vi "ETH 6 Main.vi"(7 "ETH6 Q":refnum<queue>, 8 "error in (no error)":errorcluster, 11 "connection ID":refnum<k5>) -> (0 "error out 2":errorcluster, 3 "connection ID 2":refnum<k5>)   [LabVIEW 2022 SP3]
panel:
  in  "data in":string
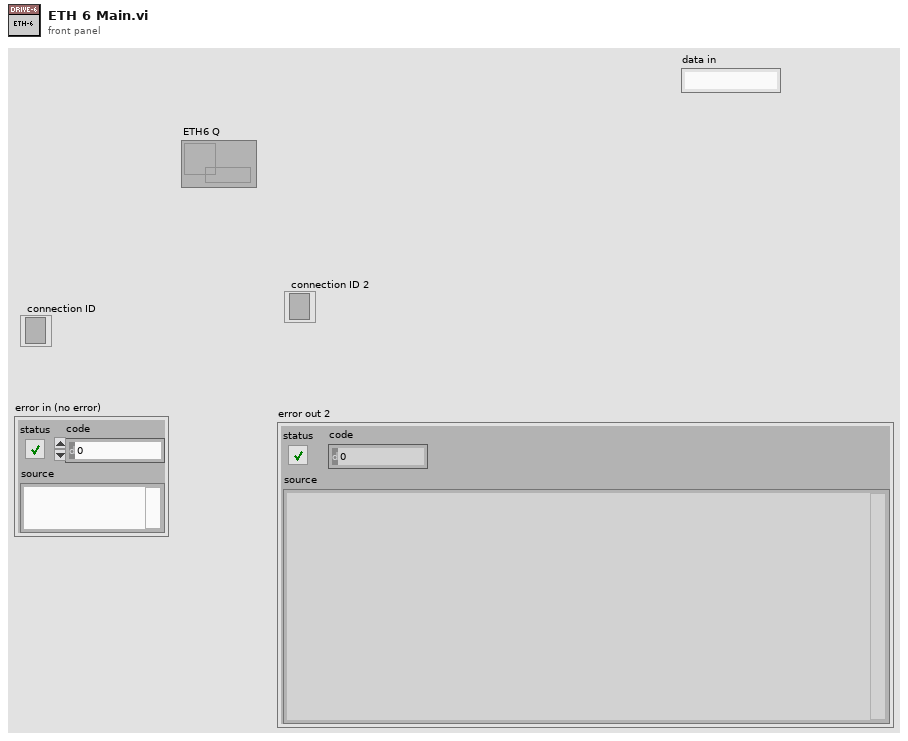
[diagram p1: front panel]
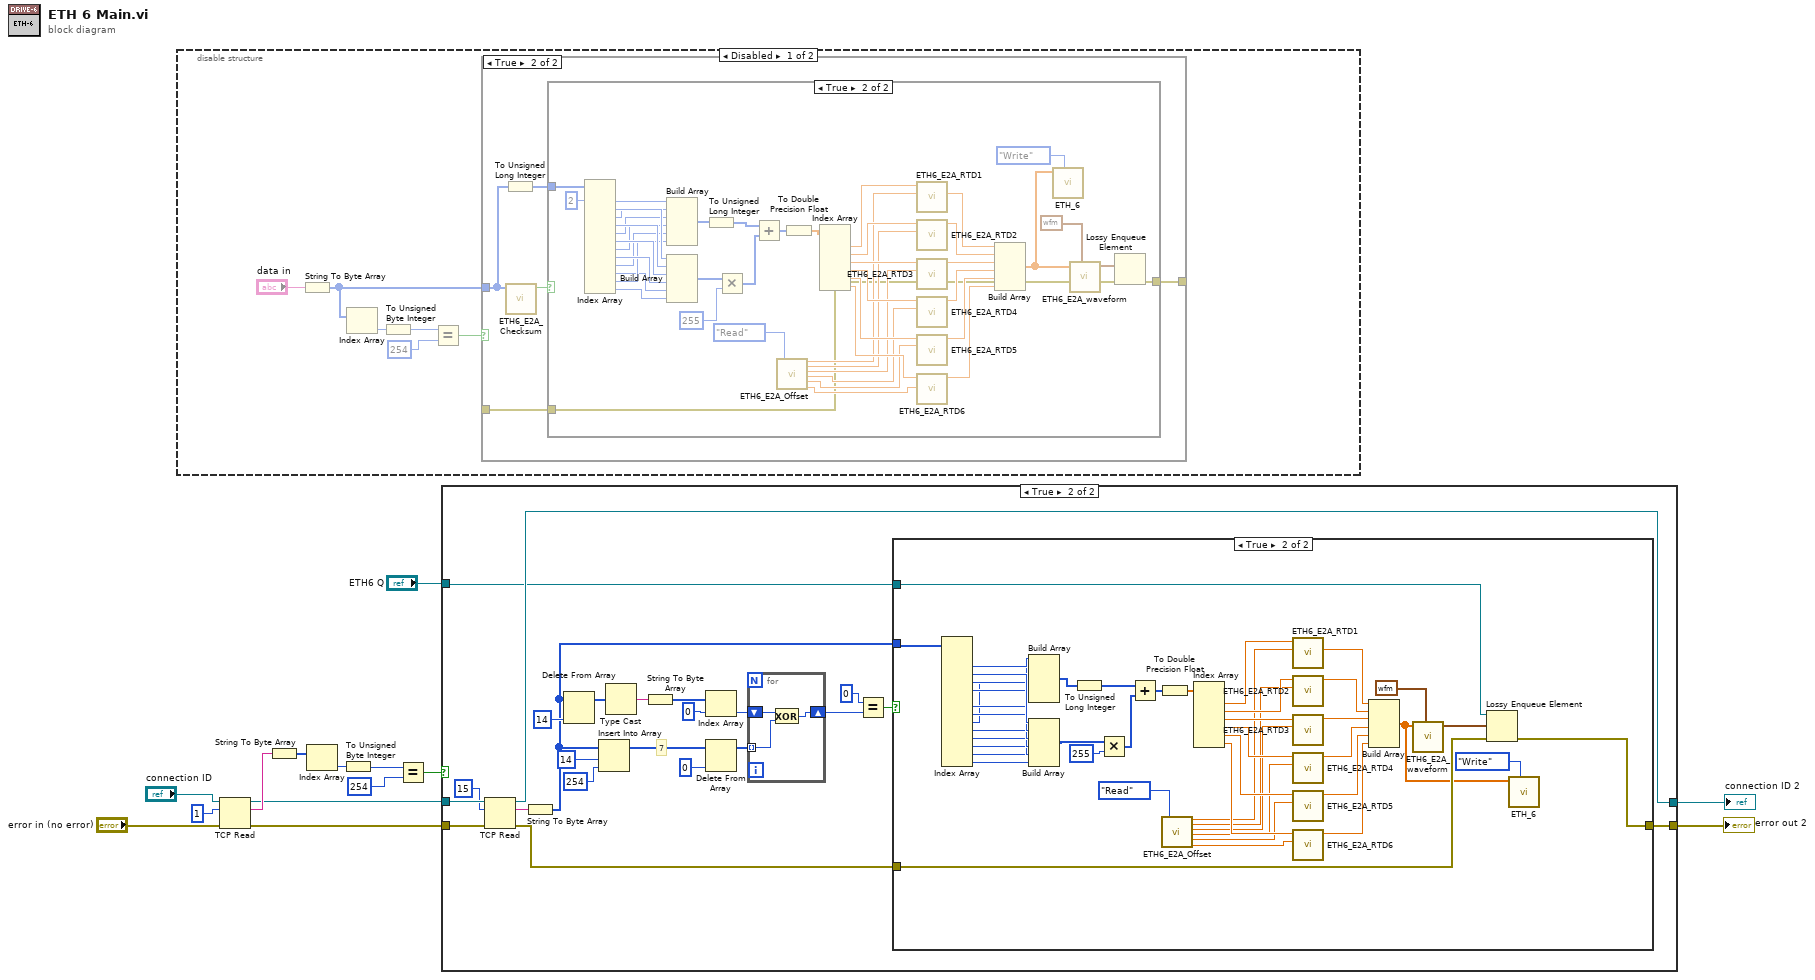
[diagram p0: block diagram]
diagram:
  n1 = disable-structure shown="Disabled" {
    frame Disabled {
      n2 = String To Byte Array(string="data in") -> (unsigned byte array=w15:u8[])
      n3 = Index Array(array=w15) -> (element=w20:u8)  [unwired: 1 in]
      n4 = To Unsigned Byte Integer(number=w20) -> (unsigned 8bit integer=w19:u8)
      n5 = Equal?(x=w19, y=u8 254) -> (x = y?=w16:bool)
      n6 = case shown="True" w16 {
        tunnel: w15 -> [_ w25]
        tunnel: _ -> [w21 w23]
        tunnel: [w21 w22] -> _
        frame False {
        }
        frame True {
          n7 = To Unsigned Long Integer(number=w25) -> (unsigned 32bit integer=w24:u32[])
          n8 = call "ETH6_E2A_Checksum.vi"("unsigned byte array"=w25) -> ("Checksum"=w26:bool)  [unwired: 10 in]
          n9 = case shown="True" w26 {
            tunnel: w24 -> [_ w29]
            tunnel: w23 -> [w27 w52]
            tunnel: [w27 w51] -> w22
            frame False {
            }
            frame True {
              n10 = Index Array(array=w29, index #1=2 ("index")) -> (element #1=w46:u32, element #2=w45:u32, element #3=w44:u32, element #4=w43:u32, element #5=w42:u32, element #6=w41:u32, element #7=w40:u32, element #8=w39:u32, element #9=w38:u32, element #10=w35:u32, element #11=w37:u32, element #12=w36:u32)  [unwired: 11 in]
              n11 = Build Array(w46, w44, w42, w40, w38, w37) -> (w47:u32[])
              n12 = Build Array(w45, w43, w41, w39, w35, w36) -> (w48:u32[])
              n13 = To Unsigned Long Integer(number=w47) -> (unsigned 32bit integer=w33:u32[])
              n14 = Multiply(x=w48, y=u32 255) -> (x*y=w32:u32[])
              n15 = Add(x=w33, y=w32) -> (x+y=w34:u32[])
              n16 = call "ETH6_E2A_Offset.vi"("Write/Read"=enum16{"Write", "Read"}."Read") -> ("RTD1 Offset Out"=w66:dbl, "RTD2 Offset Out"=w65:dbl, "RTD3 Offset Out"=w64:dbl, "RTD4 Offset out"=w63:dbl, "RTD5 Offset out"=w62:dbl, "RTD6 Offset  out"=w61:dbl)  [unwired: 13 in]
              n17 = To Double Precision Float(number=w34) -> (double precision float=w28:dbl[])
              n18 = Index Array(array=w28) -> (element #1=w73:dbl, element #2=w72:dbl, element #3=w71:dbl, element #4=w70:dbl, element #5=w69:dbl, element #6=w68:dbl)  [unwired: 6 in]
              n19 = call "ETH6_E2A_RTD1.vi"("RTD 1 Off"=w66, "Input Variable"=w73) -> ("RTD Value"=w60:dbl)  [unwired: 9 in]
              n20 = call "ETH6_E2A_RTD2.vi"("RTD 2 Off"=w65, "Input Variable"=w72) -> ("RTD Value"=w59:dbl)  [unwired: 9 in]
              n21 = call "ETH6_E2A_RTD3.vi"("RTD 3 Off"=w64, "Input Variable"=w71) -> ("RTD Value"=w58:dbl)  [unwired: 9 in]
              n22 = call "ETH6_E2A_RTD4.vi"("RTD 4 Off"=w63, "Input Variable"=w70) -> ("RTD Value"=w57:dbl)  [unwired: 9 in]
              n23 = call "ETH6_E2A_RTD5.vi"("RTD 5 Off"=w62, "Input Variable"=w69) -> ("RTD Value"=w56:dbl)  [unwired: 9 in]
              n24 = call "ETH6_E2A_RTD6.vi"("RTD 6 Off"=w61, "Input Variable"=w68) -> ("RTD Value"=w55:dbl)  [unwired: 9 in]
              n25 = Build Array(w60, w59, w58, w57, w56, w55) -> (w49:dbl[])
              n26 = call "ETH_6.vi"("Enum"=enum16{"Read", "Write"}."Write", "ETH_6"=w49) -> ()  [unwired: 8 in, 2 out]
              n27 = call "ETH6_E2A_waveform.vi"("Waveform"=waveform(dbl) {"t0"=timestamp(0 s since 1904-01-01), "dt"=0.001, "Y"=[]}, "Array in"=w49) -> ("Array out"=w53:waveform(dbl)[])  [unwired: 9 in]
              n28 = Lossy Enqueue Element(element=w53, error in (no error)=w52) -> (error out=w51:errorcluster)  [unwired: 1 in, 3 out]
            }
          }
        }
      }
    }
    frame Enabled {
    }
  }
  n29 = TCP Read(connection ID="connection ID", bytes to read=1, error in (no error)="error in (no error)") -> (connection ID out=w8:refnum<k5>, data out=w9:string, error out=w6:errorcluster)  [unwired: 2 in]
  n30 = String To Byte Array(string=w9) -> (unsigned byte array=w13:u8[])
  n31 = Index Array(array=w13) -> (element=w12:u8)  [unwired: 1 in]
  n32 = To Unsigned Byte Integer(number=w12) -> (unsigned 8bit integer=w11:u8)
  n33 = Equal?(x=w11, y=u8 254) -> (x = y?=w7:bool)
  n34 = case shown="True" w7 {
    tunnel: w8 -> [w74 w98]
    tunnel: w6 -> [w75 w97]
    tunnel: [w75 w79] -> w4
    tunnel: [w74 w96] -> w3
    tunnel: "ETH6 Q" -> [_ w76]
    frame False {
    }
    frame True {
      # "7"
      n35 = TCP Read(connection ID=w98, bytes to read=15, error in (no error)=w97) -> (connection ID out=w96:refnum<k5>, data out=w95:string, error out=w78:errorcluster)  [unwired: 2 in]
      n36 = String To Byte Array(string=w95) -> (unsigned byte array=w77:u8[])
      n37 = Delete From Array(array=w77, index=14) -> (array with subset deleted=w86:u8[])  [unwired: 1 in, 1 out]
      n38 = Insert Into Array(array=w77, index=14, new element=u8 254 ("new element/subarray")) -> (w83:u8[])
      n39 = Type Cast(x=w86) -> (*(type *) &x=w92:string)  [unwired: 1 in]
      n40 = String To Byte Array(string=w92) -> (unsigned byte array=w87:u8[])
      n41 = Index Array(array=w87, index=0) -> (element=w90:u8)
      n42 = Delete From Array(array=w83, index=0) -> (array with subset deleted=w89:u8[])  [unwired: 1 in, 1 out]
      n43 = for {
        shift-right: [w147] -> w81
        shift-left: w90 -> [w148]
        tunnel: w89 -> [w146] mode=indexing
        n44 = Exclusive Or(1:w146, 2:w148) -> (0:w147:u8)
      }
      n45 = Equal?(x=u8 0, y=w81) -> (x = y?=w80:bool)
      n46 = case shown="True" w80 {
        tunnel: w77 -> [_ w137]
        tunnel: w76 -> [_ w140]
        tunnel: w78 -> [w99 w139]
        tunnel: [w99 w138] -> w79
        frame False {
        }
        frame True {
          n47 = Index Array(array=w137) -> (element #2=w134:u8, element #3=w133:u8, element #4=w132:u8, element #5=w131:u8, element #7=w130:u8, element #8=w129:u8, element #9=w128:u8, element #10=w127:u8, element #11=w126:u8, element #12=w125:u8, element #13=w124:u8, element #14=w123:u8)  [unwired: 14 in, 2 out]
          n48 = Build Array(w134, w132, w130, w128, w126, w124) -> (w136:u8[])
          n49 = Build Array(w133, w131, w129, w127, w125, w123) -> (w135:u8[])
          n50 = To Unsigned Long Integer(number=w136) -> (unsigned 32bit integer=w142:u32[])
          n51 = Multiply(x=w135, y=u32 255) -> (x*y=w144:u32[])
          n52 = Add(x=w142, y=w144) -> (x+y=w141:u32[])
          n53 = To Double Precision Float(number=w141) -> (double precision float=w145:dbl[])
          n54 = call "ETH6_E2A_Offset.vi"("Write/Read"=enum16{"Write", "Read"}."Read") -> ("RTD1 Offset Out"=w114:dbl, "RTD2 Offset Out"=w113:dbl, "RTD3 Offset Out"=w112:dbl, "RTD4 Offset out"=w111:dbl, "RTD5 Offset out"=w110:dbl, "RTD6 Offset  out"=w109:dbl)  [unwired: 13 in]
          n55 = Index Array(array=w145) -> (element #1=w120:dbl, element #2=w119:dbl, element #3=w118:dbl, element #4=w117:dbl, element #5=w116:dbl, element #6=w115:dbl)  [unwired: 6 in]
          n56 = call "ETH6_E2A_RTD1.vi"("RTD 1 Off"=w114, "Input Variable"=w120) -> ("RTD Value"=w108:dbl)  [unwired: 9 in]
          n57 = call "ETH6_E2A_RTD2.vi"("RTD 2 Off"=w113, "Input Variable"=w119) -> ("RTD Value"=w107:dbl)  [unwired: 9 in]
          n58 = call "ETH6_E2A_RTD3.vi"("RTD 3 Off"=w112, "Input Variable"=w118) -> ("RTD Value"=w106:dbl)  [unwired: 9 in]
          n59 = call "ETH6_E2A_RTD4.vi"("RTD 4 Off"=w111, "Input Variable"=w117) -> ("RTD Value"=w105:dbl)  [unwired: 9 in]
          n60 = call "ETH6_E2A_RTD5.vi"("RTD 5 Off"=w110, "Input Variable"=w116) -> ("RTD Value"=w104:dbl)  [unwired: 9 in]
          n61 = call "ETH6_E2A_RTD6.vi"("RTD 6 Off"=w109, "Input Variable"=w115) -> ("RTD Value"=w103:dbl)  [unwired: 9 in]
          n62 = Build Array(w108, w107, w106, w105, w104, w103) -> (w102:dbl[])
          n63 = call "ETH6_E2A_waveform.vi"("Waveform"=waveform(dbl) {"t0"=timestamp(0 s since 1904-01-01), "dt"=0.001, "Y"=[]}, "Array in"=w102) -> ("Array out"=w100:waveform(dbl)[])  [unwired: 9 in]
          n64 = Lossy Enqueue Element(queue=w140, element=w100, error in (no error)=w139) -> (error out=w138:errorcluster)  [unwired: 3 out]
          n65 = call "ETH_6.vi"("Enum"=enum16{"Read", "Write"}."Write", "ETH_6"=w102) -> ()  [unwired: 8 in, 2 out]
        }
      }
    }
  }
  "error out 2" <- w4
  "connection ID 2" <- w3
